vi "complementary_color.vi"(1 "color in":u32(colorbox)=29532) -> (0 "complementary color out":u32(colorbox))   [LabVIEW 2010]
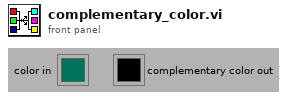
[diagram p1: front panel]
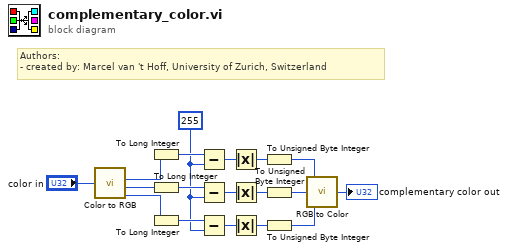
[diagram p0: block diagram]
diagram:
  w9 = 255
  # "Authors: \n- created by: Marcel van 't Hoff, University of Zurich, Switzerland"
  n1 = call <vilib>:"Color to RGB.vi"("Color"="color in") -> ("R"=w13:u8, "G"=w17:u8, "B"=w12:u8)  [unwired: 1 out]
  n2 = To Long Integer(number=w13) -> (32bit integer=w11:i32)
  n3 = To Long Integer(number=w17) -> (32bit integer=w15:i32)
  n4 = To Long Integer(number=w12) -> (32bit integer=w10:i32)
  n5 = Subtract(x=w11, y=w9) -> (x-y=w7:i32)
  n6 = Subtract(x=w15, y=w9) -> (x-y=w16:i32)
  n7 = Subtract(x=w10, y=w9) -> (x-y=w14:i32)
  n8 = Absolute Value(x=w7) -> (abs(x)=w8:i32)
  n9 = Absolute Value(x=w16) -> (abs(x)=w4:i32)
  n10 = Absolute Value(x=w14) -> (abs(x)=w5:i32)
  n11 = To Unsigned Byte Integer(number=w8) -> (unsigned 8bit integer=w6:u8)
  n12 = To Unsigned Byte Integer(number=w4) -> (unsigned 8bit integer=w3:u8)
  n13 = To Unsigned Byte Integer(number=w5) -> (unsigned 8bit integer=w2:u8)
  n14 = call <vilib>:"RGB to Color.vi"("B"=w2, "G"=w3, "R"=w6) -> ("Color"=→"complementary color out":u32)
